vi "Write Elevator State Ref.vi"(8 "error in (no error)":errorcluster, 10 "Elevator State Ref":refnum<vi>, 11 "Elevator State Receiver in":refnum<class "Elevator State Receiver.lvclass">) -> (0 "error out":errorcluster, 3 "Elevator State Receiver out":refnum<class "Elevator State Receiver.lvclass">)   [LabVIEW 2014, in "Elevator.lvlib" / "Elevator State Receiver.lvclass"]
uses:
  Elevator State Receiver.lvclass
  Elevator Class/Elevator State.ctl
  Elevator State Receiver.lvclass/Elevator State Receiver.ctl
  Elevator Class/Elevator.lvclass
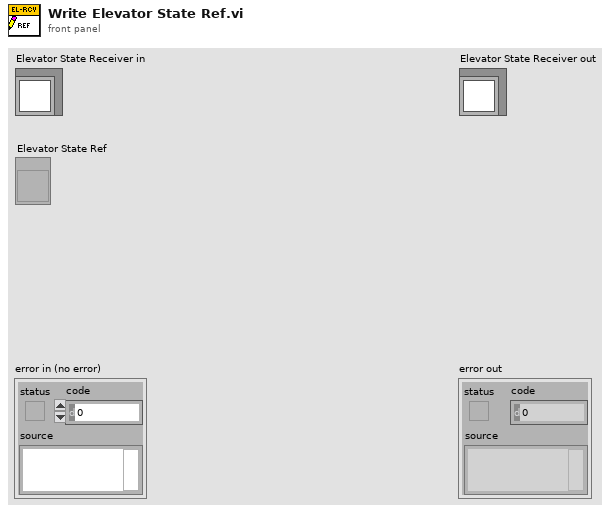
[diagram p1: front panel]
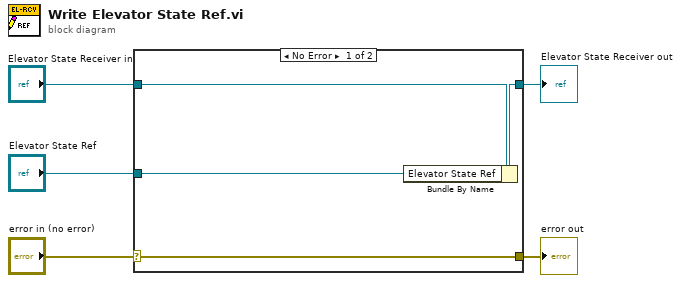
[diagram p0: block diagram]
diagram:
  n1 = case shown="No Error" "error in (no error)" {
    selector: "error in (no error)" -> [w9 w10]
    tunnel: [w9 w10] -> w4
    tunnel: [w7 w11] -> w2
    tunnel: "Elevator State Receiver in" -> [w8 w11]
    tunnel: "Elevator State Ref" -> [w6 _]
    frame No Error {
      n2 = Bundle By Name(cluster=w8, "Elevator State Ref"=w6) -> (w7:refnum<class "Elevator State Receiver.lvclass">)
    }
    frame Error {
    }
  }
  "error out" <- w4
  "Elevator State Receiver out" <- w2
